vi "Download Waveforms.vi"(0 "fpga interface in":refnum<k20>, 5 "stream instance":i32, 7 "waveforms":waveform(dbl)[](array[waveform]), 11 "error in":errorcluster) -> (4 "fpga interface out":refnum<k20>, 6 "stream instance out":i32, 15 "error out":errorcluster)   [LabVIEW 2018, in "GettingStarted_5745_Host.lvlib"]
uses:
  GettingStarted_5745_Host.lvlib
  <vilib>/rvi/interface/nirviMethod/nirviMethod.xnode
  <vilib>/rvi/interface/nirviReadWriteControl/nirviReadWriteControl.xnode
  <resource>/objmgr/niflexrioapiChannel.rc
  <instrlib>/FlexRIO/API/Host/v1/NI FlexRIO API v1.lvlib
  <vilib>/Utility/error.llb/Error Cluster From Error Code.vi
  <vilib>/rvi/interface/Simulation/niFpgaSimulationCallBeginRW.vi
  <vilib>/rvi/errors/niLvFpgaAdjustHostInterfaceError.vi
  NiFpgaLv.dll
  <instrlib>/FlexRIO/API/Host/v1/NI FlexRIO/API/Get Property Reference - Fpga Small.vi
  <vilib>/FPGAPlugInAG/Dynamic/niLvFpga_WriteFifo_Dynamic.vi
  <vilib>/rvi/errors/niLvFpgaMergeErrorWithErrorCode.vi
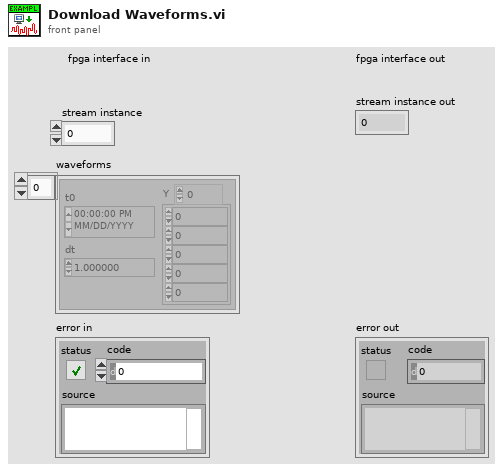
[diagram p1: front panel]
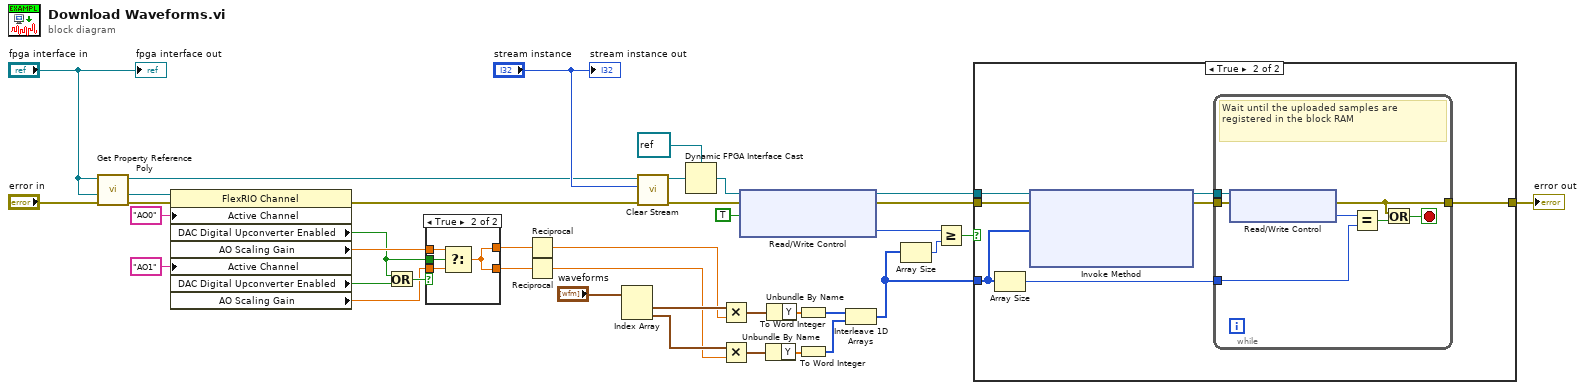
[diagram p0: block diagram]
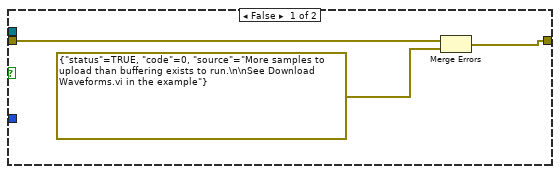
[diagram p3: hidden frame]
diagram:
  n1 = call-poly <instrlib>:"Get Property Reference Poly.vi"("error in (no error)"="error in", "fpga interface in"="fpga interface in") -> ("error out"=w3:errorcluster, "property reference"=w2:refnum<k20>)  [unwired: 4 in, 1 out]
  n2 = property class="FlexRIO Channel"(reference=w2, error in=w3, "Active Channel"="AO0", "Active Channel"="AO1") -> (error out=w1:errorcluster, "DAC Digital Upconverter Enabled"=w6:bool, "AO Scaling Gain"=w8:dbl, "DAC Digital Upconverter Enabled"=w9:bool, "AO Scaling Gain"=w7:dbl)  [unwired: 1 out]
  n3 = Or(x=w6, y=w9) -> (x .or. y?=w10:bool)
  n4 = case shown="True" w10 {
    tunnel: w8 -> [w40 w43]
    tunnel: w7 -> [w39 w42]
    tunnel: [w40 w41] -> w4
    tunnel: [w39 w41] -> w5
    tunnel: w6 -> [_ w44]
    frame False {
    }
    frame True {
      n5 = Select(t=w43, s=w44, f=w42) -> (s? t:f=w41:dbl)
    }
  }
  n6 = Reciprocal(x=w4) -> (1/x=w23:dbl)
  n7 = Reciprocal(x=w5) -> (1/x=w22:dbl)
  n8 = Index Array(array="waveforms") -> (element #1=w35:waveform(dbl), element #2=w34:waveform(dbl))  [unwired: 2 in]
  n9 = call <instrlib>:"Clear Stream.vi"("error in (no error)"=w1, "stream index"="stream instance", "refnum in"="fpga interface in") -> ("error out"=w27:errorcluster, "refnum out"=w19:refnum<k20>)  [unwired: 7 in]
  n10 = Dynamic FPGA Interface Cast(Session In=refnum<k20> refnum ("fpga interface in"), Type=w19) -> (Session Out=w18:refnum<k20>)
  n11 = Multiply(x=w35, y=w23) -> (x*y=w38:waveform(dbl))
  n12 = Multiply(x=w34, y=w22) -> (x*y=w37:waveform(dbl))
  n13 = xnode "Read/Write Control"("FPGA VI Reference In"=w18, "error in"=w27, "reset circular buffer"=TRUE) -> ("FPGA VI Reference Out"=w29:refnum<k20>, "error out"=w28:errorcluster, "buffer size in elements"=w13:u64)
  n14 = Unbundle By Name(w37) -> ("Y"=w24:dbl[])
  n15 = Unbundle By Name(w38) -> ("Y"=w25:dbl[])
  n16 = To Word Integer(number=w25) -> (16bit integer=w33:i16[])
  n17 = To Word Integer(number=w24) -> (16bit integer=w32:i16[])
  n18 = Interleave 1D Arrays(w33, w32) -> (w17:i16[])
  n19 = Array Size(array=w17) -> (size(s)=w14:i32)
  n20 = Greater Or Equal?(x=w13, y=w14) -> (x >= y?=w15:bool)
  n21 = case shown="True" w15 {
    tunnel: w29 -> [_ w54]
    tunnel: w28 -> [w47 w53]
    tunnel: w17 -> [_ w49]
    tunnel: [w45 w50] -> w16
    frame False {
      n22 = Merge Errors(w47, errorcluster {"status"=TRUE, "code"=0, "source"="More samples to upload than buffering exists to run.\n\nSee Download Waveforms.vi in the example"} ("error in")) -> (w45:errorcluster)
    }
    frame True {
      n23 = Array Size(array=w49) -> (size(s)=w48:i32)
      n24 = xnode "Invoke Method"("FPGA VI Reference In"=w54, "error in"=w53, "Data"=w49) -> ("FPGA VI Reference Out"=w52:refnum<k20>, "error out"=w51:errorcluster)  [unwired: 1 in, 1 out]
      n25 = while {
        tunnel: w52 -> [w61]
        tunnel: w51 -> [w60]
        tunnel: w48 -> [w58]
        tunnel: [w56] -> w50
        stop <- w57 stop-if-true
        # "Wait until the uploaded samples are registered in the block RAM"
        n26 = xnode "Read/Write Control"("FPGA VI Reference In"=w61, "error in"=w60) -> ("error out"=w56:errorcluster, "written elements"=w59:u64)  [unwired: 1 out]
        n27 = Equal?(x=w59, y=w58) -> (x = y?=w55:bool)
        n28 = Or(x=w56, y=w55) -> (x .or. y?=w57:bool)
      }
    }
  }
  "error out" <- w16
  "fpga interface out" <- "fpga interface in"
  "stream instance out" <- "stream instance"
